vi "Configure Eye Diagram.vi"(6 "Eye Y Resolution (0: er128)":i32(ring) items=["er128", "er256", "er512", "er1024"], 7 "Eye X Resolution (0: er128)":i32(ring) items=["er128", "er256", "er512", "er1024"], 8 "error in (no error)":errorcluster, 9 "Number Of Eyes (2)":i32=2, 10 "Calculate Eye Diagram (T: Enable)":bool=TRUE, 11 "VISA resource name":refnum<visa-resource-name>) -> (0 "error out":errorcluster, 3 "VISA resource name out":refnum<visa-resource-name>)   [LabVIEW 2014, in "Stanford Research SR1.lvlib"]
doc: "Configures the attributes of the Eye Diagram."
uses:
  Stanford Research SR1.lvlib
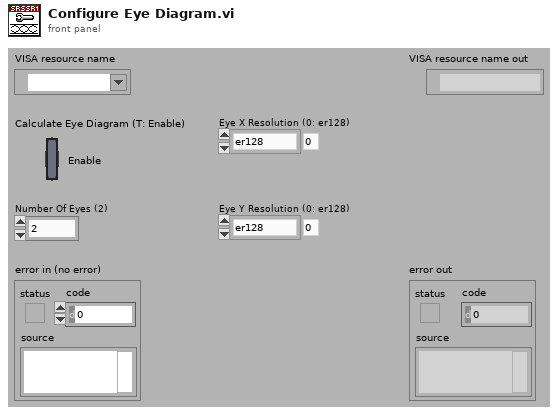
[diagram p1: front panel]
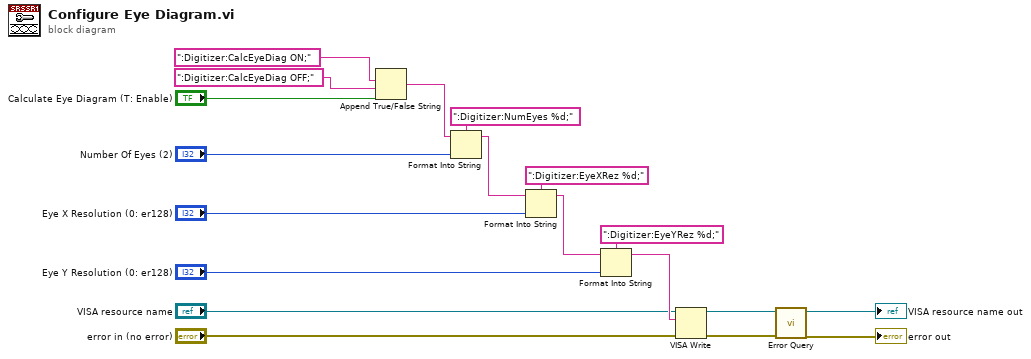
[diagram p0: block diagram]
diagram:
  n1 = Append True/False String(1:"Calculate Eye Diagram (T: Enable)", 2:":Digitizer:CalcEyeDiag OFF;", 3:":Digitizer:CalcEyeDiag ON;") -> (0:w16:string)  [unwired: 1 in]
  n2 = Format Into String(format string=":Digitizer:NumEyes %d;", initial string=w16, "Number Of Eyes (2)") -> (resulting string=w13:string)  [unwired: 1 in, 1 out]
  n3 = Format Into String(format string=":Digitizer:EyeXRez %d;", initial string=w13, "Eye X Resolution (0: er128)") -> (resulting string=w10:string)  [unwired: 1 in, 1 out]
  n4 = Format Into String(format string=":Digitizer:EyeYRez %d;", initial string=w10, "Eye Y Resolution (0: er128)") -> (resulting string=w7:string)  [unwired: 1 in, 1 out]
  n5 = VISA Write(VISA resource name="VISA resource name", write buffer=w7, error in (no error)="error in (no error)") -> (VISA resource name out=w4:refnum<visa-resource-name>, error out=w3:errorcluster)  [unwired: 1 out]
  n6 = call "Error Query.vi"("error in (no error)"=w3, "VISA resource name"=w4) -> ("error out"=→"error out":errorcluster, "VISA resource name out"=→"VISA resource name out":refnum<visa-resource-name>)  [unwired: 6 in, 2 out]
